vi "Is Authenticated.vi"(11 "Session.lvclass":refnum<class "Session.lvclass">) -> (3 "Authenticated":bool)   [LabVIEW 2026, in "Session.lvclass"]
uses:
  Session.lvclass
  Session.lvclass/Session.ctl
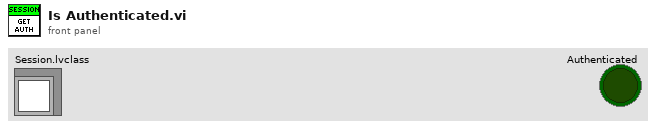
[diagram p1: front panel]
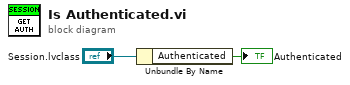
[diagram p0: block diagram]
diagram:
  n1 = Unbundle By Name("Session.lvclass") -> ("Authenticated"=→"Authenticated":bool)
